vi "skipMatColRow.vi"(8 "error in (no error)":errorcluster, 9 "Skip Col Idx":i32[](array[numeric]), 10 "Skip Row Idx":i32[](array[numeric]), 11 "Matrix":dbl[][](array[numeric])) -> (0 "error out":errorcluster, 3 "Sub-Array":dbl[][](array[numeric]))   [LabVIEW 2016]
doc: "Skip the rows or columns in a matrix."
uses:
  getSubArray2D.vi
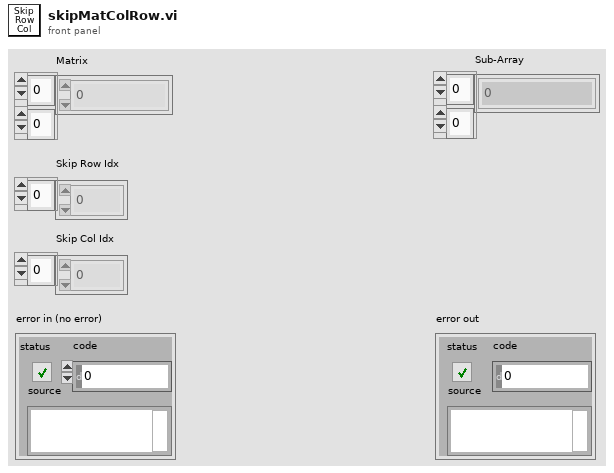
[diagram p1: front panel]
types:
  T1 = cluster{"Non-Overlap Idx Array":i32[], "Non-Overlap Idx Array":i32[]}
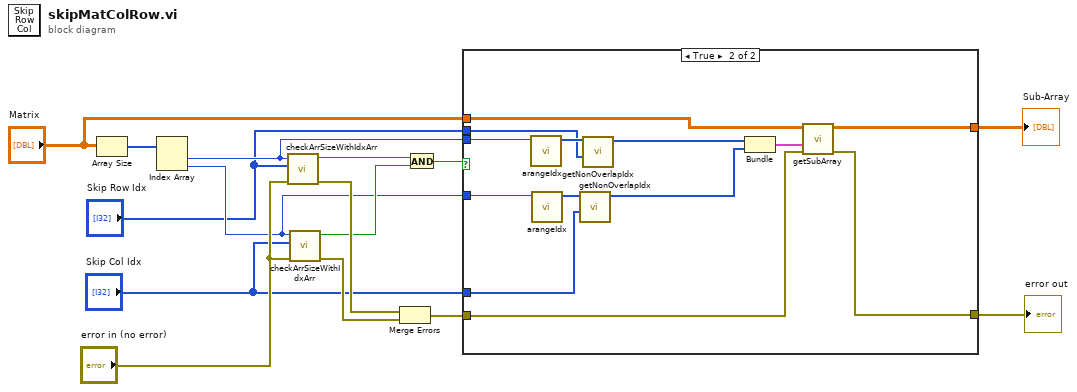
[diagram p0: block diagram]
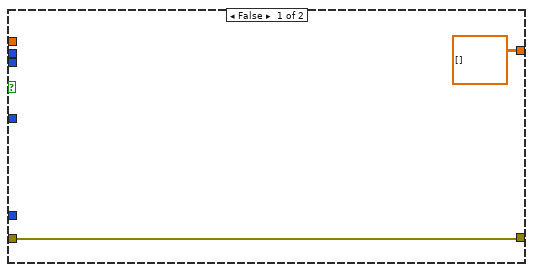
[diagram p2: hidden frame]
diagram:
  n1 = Array Size(array="Matrix") -> (size(s)=w15:i32[])
  n2 = Index Array(array=w15) -> (element #1=w8:i32, element #2=w7:i32)  [unwired: 2 in]
  n3 = call "checkArrSizeWithIdxArr.vi"("error in (no error)"="error in (no error)", "Idx Array"="Skip Row Idx", "Array Size"=w8) -> ("error out"=w13:errorcluster, "In Spec"=w11:bool)  [unwired: 7 in]
  n4 = call "checkArrSizeWithIdxArr.vi"("error in (no error)"="error in (no error)", "Idx Array"="Skip Col Idx", "Array Size"=w7) -> ("error out"=w12:errorcluster, "In Spec"=w10:bool)  [unwired: 7 in]
  n5 = Merge Errors(w13, w12) -> (w6:errorcluster)
  n6 = And(x=w11, y=w10) -> (x .and. y?=w9:bool)
  n7 = case shown="True" w9 {
    tunnel: w8 -> [_ w25]
    tunnel: w7 -> [_ w24]
    tunnel: w6 -> [w16 w21]
    tunnel: "Skip Row Idx" -> [_ w23]
    tunnel: "Skip Col Idx" -> [_ w22]
    tunnel: "Matrix" -> [_ w20]
    tunnel: [w16 w19] -> w3
    tunnel: [dbl[][] [] ("Sub-Array") w18] -> w2
    frame False {
    }
    frame True {
      n8 = call "arangeIdx.vi"("Number"=w25) -> ("Idx Array"=w26:i32[])  [unwired: 10 in]
      n9 = call "arangeIdx.vi"("Number"=w24) -> ("Idx Array"=w27:i32[])  [unwired: 10 in]
      n10 = call "getNonOverlapIdx.vi"("Input Idx Array"=w27, "Overlap Idx Array"=w22) -> ("Non-Overlap Idx Array"=w29:i32[])  [unwired: 8 in]
      n11 = call "getNonOverlapIdx.vi"("Input Idx Array"=w26, "Overlap Idx Array"=w23) -> ("Non-Overlap Idx Array"=w28:i32[])  [unwired: 8 in]
      n12 = Bundle("Non-Overlap Idx Array"=w28, "Non-Overlap Idx Array"=w29) -> (w30:T1)  [unwired: 1 in]
      n13 = call-poly "getSubArray.vi"("error in (no error)"=w21, "Index Array Cluster"=w30, "2D Array"=w20) -> ("error out"=w19:errorcluster, "Sub-Array"=w18:dbl[][])  [unwired: 7 in]
    }
  }
  "Sub-Array" <- w2
  "error out" <- w3
